vi "Select Model.vi"() -> (1 "Cancel out":bool, 3 "Model out":string)   [LabVIEW 2017]
uses:
  Controls/Logging FGV.ctl
panel:
  in  "New Shift":bool
  out "Reject Count":u32
  out "Total Count":u32
  out "OEE 2":T1 caption="Latest Measurements" {"AVL" format="%#.1f"; "PRF" format="%#.1f"; "QUA" format="%#.1f"; "OEE" format="%#.1f"}
  out "Timestamp":string caption="Start Time"
  out "PDT (Hr)":dbl caption="Planned Down Time (Hours)"
  out "SPT (Hr)":dbl caption="Scheduled Production Time (Hours)"
  in  "Model":string(combo)="Model A:188.9"
  in  "Cancel Button":bool
  in  "Continue":bool
  # "Please select the Model that you wish to run"
  # "Previous Shift Information"
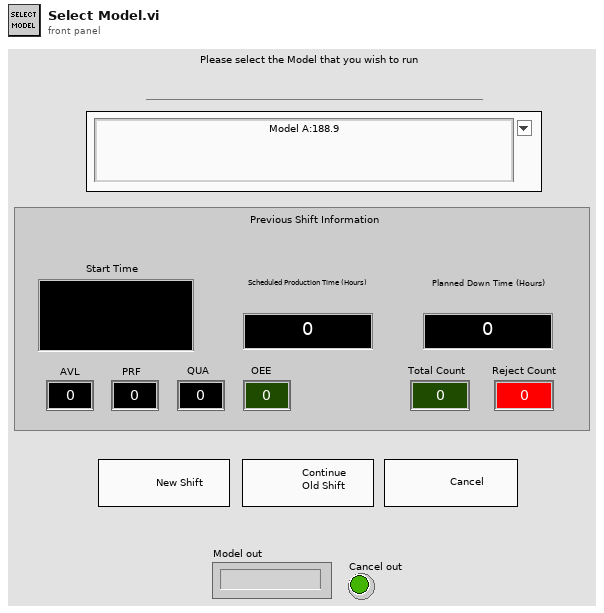
[diagram p1: front panel]
types:
  T1 = cluster{"AVL":dbl, "PRF":dbl, "QUA":dbl, "OEE":dbl}
  T2 = typedef "Logging FGV.ctl" = enum16{"Start Shift", "Log Index", "Read Shift", "Close Shift"}
  T3 = cluster{"Time-Stamp":timestamp, "Scheduled Time":dbl, "Planned Downtime":dbl}
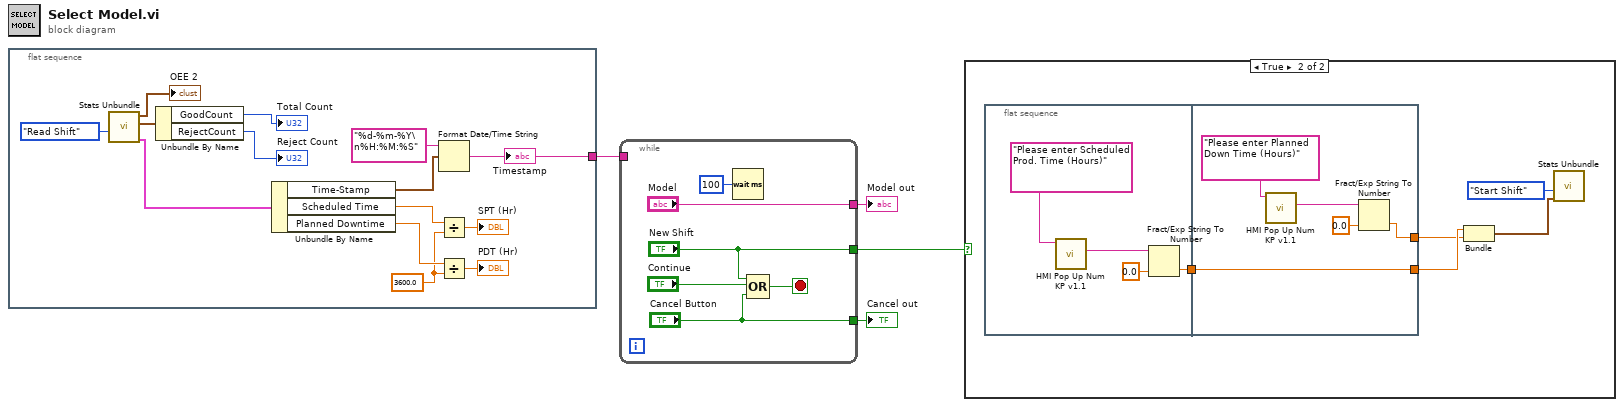
[diagram p0: block diagram]
diagram:
  n1 = flat-sequence {
    tunnel: [w9] -> w2
    frame #0 {
      w14 = 3600.0 ("y")
      n2 = call "Stats Unbundle.vi"("State"=Logging_FGV."Read Shift") -> ("NAT Cluster out"=w17:T3, "Counters"=w8:cluster{"GoodCount":u32, "RejectCount":u32}, "OEE Cluster"=→"OEE 2":T1)  [unwired: 6 in, 2 out]
      n3 = Unbundle By Name(w8) -> ("GoodCount"=→"Total Count":u32, "RejectCount"=→"Reject Count":u32)
      n4 = Unbundle By Name(w17) -> ("Time-Stamp"=w10:timestamp, "Scheduled Time"=w16:dbl, "Planned Downtime"=w15:dbl)
      n5 = Format Date/Time String(time format string (%c)="%d-%m-%Y\n%H:%M:%S", seconds (now)=w10) -> (date/time string=w9:string)  [unwired: 1 in]
      "Timestamp" <- w9
      n6 = Divide(x=w16, y=w14) -> (x/y=→"SPT (Hr)":dbl)
      n7 = Divide(x=w15, y=w14) -> (x/y=→"PDT (Hr)":dbl)
    }
  }
  n8 = while {
    tunnel: ["Model"] -> w4
    tunnel: ["Cancel Button"] -> w3
    tunnel: ["New Shift"] -> w1
    tunnel: w2 -> [_]
    stop <- w23 stop-if-true
    n9 = Wait (ms)(milliseconds to wait=u32 100) -> ()  [unwired: 1 out]
    n10 = Compound Arithmetic op=OR("New Shift", "Continue", "Cancel Button") -> (w23:bool)
  }
  "Model out" <- w4
  "Cancel out" <- w3
  n11 = case shown="True" w1 {
    frame False {
    }
    frame True {
      n12 = flat-sequence {
        tunnel: [w30] -> w29
        tunnel: [w35] -> w27
        tunnel: w29 -> [w35]
        tunnel: [w34] -> w25
        frame #0 {
          n13 = call "HMI Pop Up Num KP v1.1.vi"("Message In"="Please enter Scheduled Prod. Time (Hours)") -> ("String Out"=w31:string)  [unwired: 9 in, 1 out]
          n14 = Fract/Exp String To Number(string=w31, default (0 dbl)=0.0 ("default (0 I32)")) -> (number=w30:dbl)  [unwired: 2 in, 1 out]
        }
        frame #1 {
          n15 = call "HMI Pop Up Num KP v1.1.vi"("Message In"="Please enter Planned Down Time (Hours)") -> ("String Out"=w38:string)  [unwired: 9 in, 1 out]
          n16 = Fract/Exp String To Number(string=w38, default (0 dbl)=0.0 ("default (0 I32)")) -> (number=w34:dbl)  [unwired: 2 in, 1 out]
        }
      }
      n17 = Bundle(w27, w25) -> (w26:cluster{dbl, dbl})  [unwired: 1 in]
      n18 = call "Stats Unbundle.vi"("NAT Cluster in"=w26, "State"=Logging_FGV."Start Shift") -> ()  [unwired: 5 in, 5 out]
    }
  }
